vi "EDS Read Application.vi"(8 "error in (no error)":errorcluster) -> (0 "error out":errorcluster)   [LabVIEW 2021, in "CANOpen Addon System Explorer.lvlib"]
uses:
  CANOpen Addon System Explorer.lvlib
  Shared/SDO Parameters Array.ctl
  Shared/CANOpen_SDO Settings.ctl
  Shared/CANOpen Addon Shared.lvlib
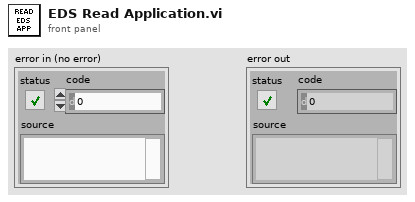
[diagram p1: front panel]
types:
  T1 = typedef "CANOpen Addon Shared.lvlib/SDO Parameters Array.ctl" = T2[]
  T2 = typedef "CANOpen Addon Shared.lvlib/CANOpen_SDO Settings.ctl" = cluster{"Object Index":u16, "Sub-Index (0)":u8, "Block Data":u8[], "Name":string}
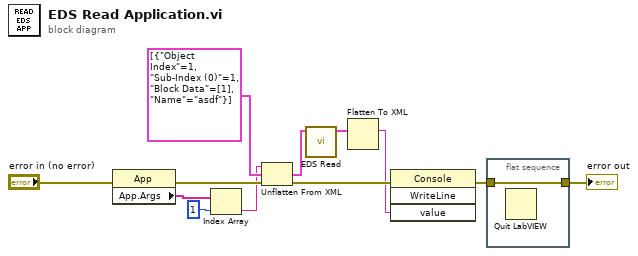
[diagram p0: block diagram]
diagram:
  n1 = property class="App"(error in="error in (no error)") -> (error out=w10:errorcluster, "App.Args"=w12:string[])  [unwired: 1 in, 1 out]
  n2 = Index Array(array=w12, index=1) -> (element=w5:string)
  n3 = Unflatten From XML(xml string=w5, type=T1 [{"Object Index"=1, "Sub-Index (0)"=1, "Block Data"=[1], "Name"="asdf"}] ("SDO Parameters"), error in (no error)=w10) -> (value=w4:T1, error out=w2:errorcluster)
  n4 = call "EDS Read.vi"("SDO Parameters"=w4) -> ("SDO Parameters out"=w3:T2[])  [unwired: 10 in]
  n5 = Flatten To XML(6:w3) -> (2:w1:string)
  n6 = invoke class="Console" method="WriteLine"(error in=w2, "value"=w1) -> (error out=w9:errorcluster)  [unwired: 2 in, 3 out]
  n7 = flat-sequence {
    tunnel: w9 -> [w13]
    tunnel: [w13] -> w8
    frame #0 {
      n8 = Quit LabVIEW() -> ()  [unwired: 1 in]
    }
  }
  "error out" <- w8
